vi "Robo Garra - Apres13.05.vi"   [LabVIEW 2016]
uses:
  <vilib>/NXT/Subs/LVHSConnector.ctl
  <vilib>/NXT/LegoClasses/BrickReference/BrickReference.lvclass
  <vilib>/NXT/Block Support/NXT_OutputPort.ctl
  <vilib>/NXT/Block Support/NXT_InputPort.ctl
  <vilib>/NXT/Block Support/NXT_ButtonSelector.ctl
  <vilib>/NXT/Dual Mode Library/Waits/Wait_Num.vi
  <vilib>/NXT/NXTIO Xnodes/NXTIONodeSubVIs/NXTMoveMotors.vi
  <vilib>/NXT/NXTIO Xnodes/NXTIONodeSubVIs/NXTStopMotors.vi
  <vilib>/NXT/Dual Mode Library/Sensors/EV3_Color_Reflect.vi
  <vilib>/NXT/Dual Mode Library/Sound/Tone.vi
  <vilib>/NXT/Dual Mode Library/Sensors/EV3_Ultrasonic_CM.vi
  <vilib>/NXT/Dual Mode Library/Sensors/readNXTButton.vi
  <vilib>/NXT/NXTIO Xnodes/AddressXNode/NXTIOAddress.xnode
  <vilib>/NXT/NXTIO Xnodes/NXTIOXNode/NXTIO.xnode
types:
  T1 = typedef "LVHSConnector.ctl" = refnum<class "BrickReference.lvclass">
  T2 = typedef "NXT_OutputPort.ctl" = u8
  T3 = typedef "NXT_ButtonSelector.ctl" = u16
  T4 = typedef "NXT_InputPort.ctl" = u32
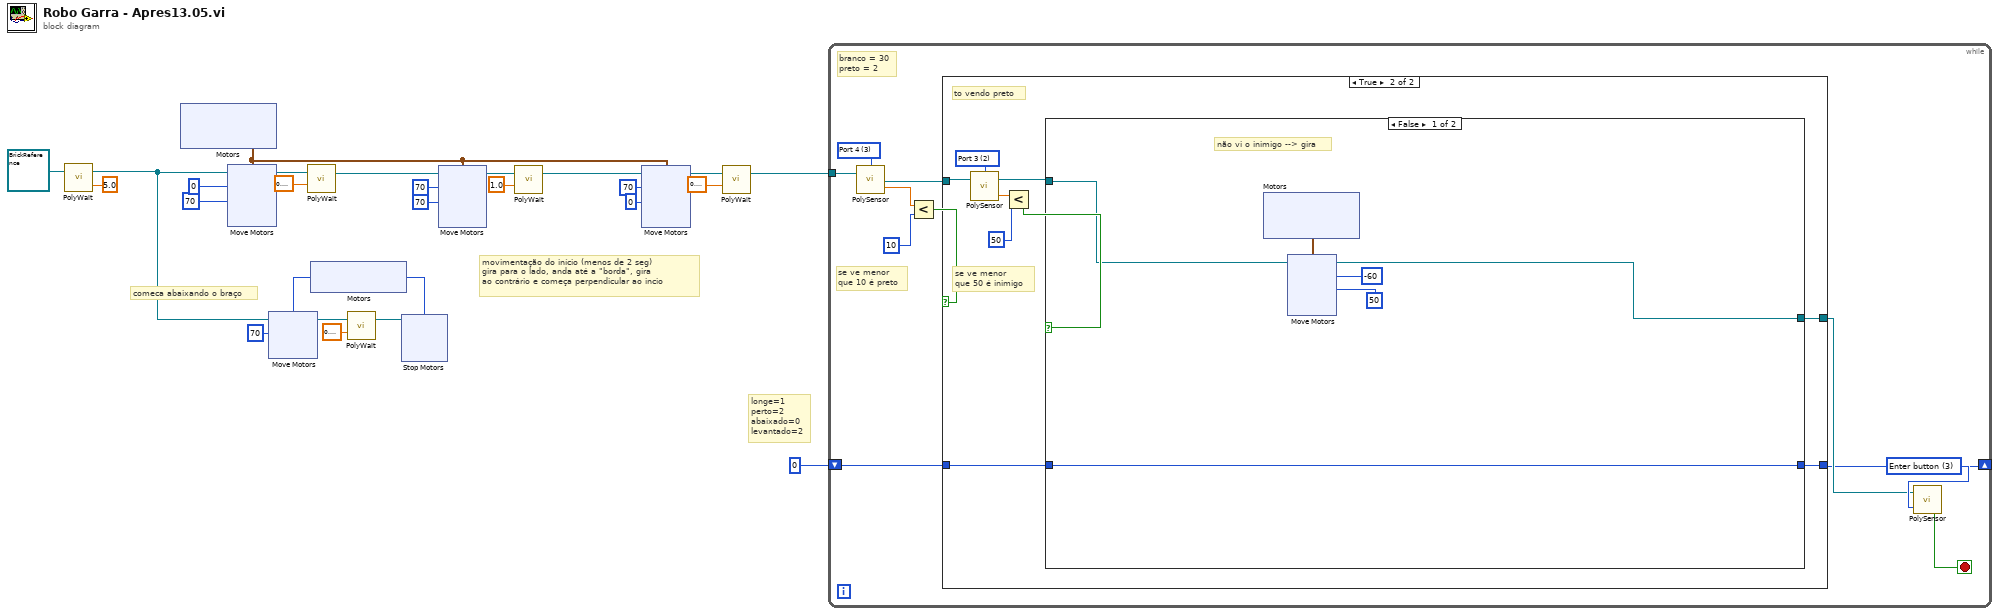
[diagram p0: block diagram]
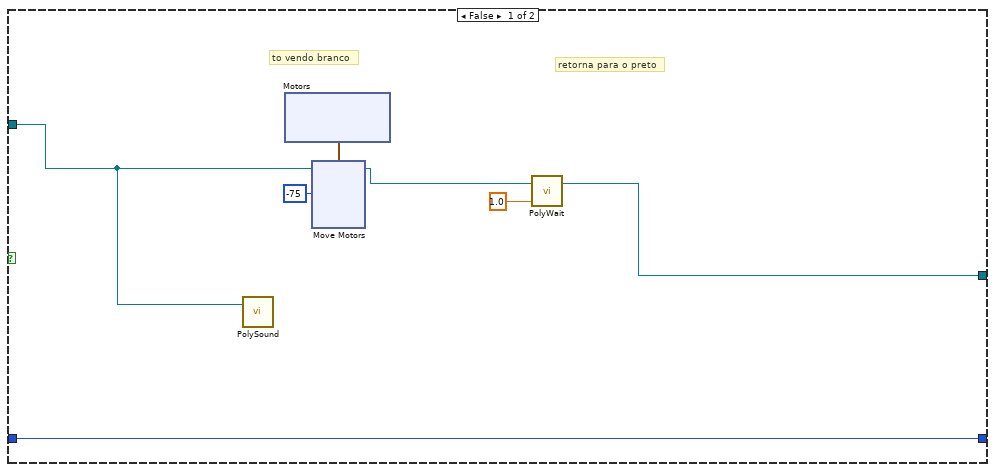
[diagram p2: hidden frame]
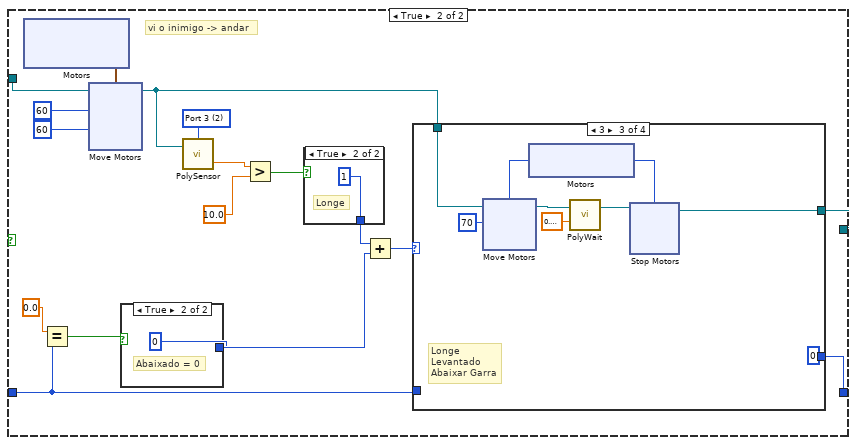
[diagram p3: hidden frame]
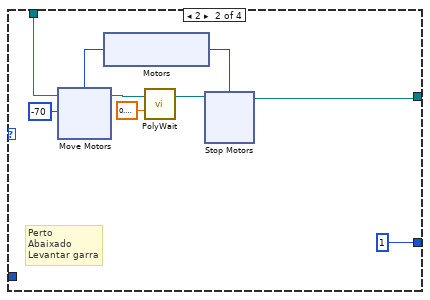
[diagram p5: hidden frame]
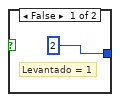
[diagram p7: hidden frame]
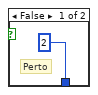
[diagram p8: hidden frame]
diagram:
  # "movimentação do início (menos de 2 seg)\ngira para o lado, anda até a \"borda\", gira \nao contrário e começa perpendicular ao incio"
  # "comeca abaixando o braço"
  # "longe=1\nperto=2\nabaixado=0\nlevantado=2"
  n1 = call-poly <vilib>:"PolyWait.vi"("Time (1 sec)"=sgl 5.0, "NXT/EV3"=T1 refnum ("y")) -> ("NXT/EV3"=w15:T1)  [unwired: 2 in]
  n2 = xnode "Motors"() -> ("Motor"=w7:cluster{"Port":T2, "Port":T2})
  n3 = xnode "Move Motors"("Power/Speed 2"=i8 70, "Power/Speed 1"=i8 0, "Motors"=w7, "NXT/EV3"=w15) -> ("NXT/EV3"=w13:T1)
  n4 = call-poly <vilib>:"PolyWait.vi"("Time (1 sec)"=sgl 0.3, "NXT/EV3"=w13) -> ("NXT/EV3"=w3:T1)  [unwired: 2 in]
  n5 = xnode "Motors"() -> ("Motor"=w19:T2)
  n6 = xnode "Move Motors"("Power/Speed 1"=i8 70, "Motors"=w19, "NXT/EV3"=w15) -> ("NXT/EV3"=w21:T1)
  n7 = call-poly <vilib>:"PolyWait.vi"("Time (1 sec)"=sgl 0.3, "NXT/EV3"=w21) -> ("NXT/EV3"=w22:T1)  [unwired: 2 in]
  n8 = xnode "Stop Motors"("Motors"=w19, "NXT/EV3"=w22) -> ()  [unwired: 1 out]
  n9 = xnode "Move Motors"("Power/Speed 2"=i8 70, "Power/Speed 1"=i8 70, "Motors"=w7, "NXT/EV3"=w3) -> ("NXT/EV3"=w10:T1)
  n10 = call-poly <vilib>:"PolyWait.vi"("Time (1 sec)"=sgl 1.0, "NXT/EV3"=w10) -> ("NXT/EV3"=w2:T1)  [unwired: 2 in]
  n11 = xnode "Move Motors"("Power/Speed 2"=i8 0, "Power/Speed 1"=i8 70, "Motors"=w7, "NXT/EV3"=w2) -> ("NXT/EV3"=w4:T1)
  n12 = call-poly <vilib>:"PolyWait.vi"("Time (1 sec)"=sgl 0.3, "NXT/EV3"=w4) -> ("NXT/EV3"=w1:T1)  [unwired: 2 in]
  n13 = while {
    tunnel: w1 -> [w35]
    shift-right: [w28] -> _
    shift-left: 0 -> [w32]
    stop <- w30 stop-if-true
    w31 = T3 3 items=["Enter button"=3, "Left button"=2, "Right button"=1, "Up Button"=4, "Down Button"=5] ("Button (Enter button)")
    w33 = T4 3 items=["Port 1", "Port 2", "Port 3", "Port 4"] ("Port (Port 1)")
    # "se ve menor \nque 10 é preto"
    # "branco = 30\npreto = 2"
    n14 = call-poly <vilib>:"PolySensor.vi"("NXT/EV3"=w35, "Port (Port 1)"=w33) -> ("Scaled Value"=w36:sgl, "NXT/EV3"=w34:T1)  [unwired: 1 in]
    n15 = Less?(x=w36, y=10) -> (x < y?=w27:bool)
    n16 = case shown="True" w27 {
      tunnel: w34 -> [w37 w61]
      tunnel: w32 -> [w38 w58]
      tunnel: [w39 w57] -> w29
      tunnel: [w38 w56] -> w28
      frame False {
        w42 = i8 -75 ("Power/Speed 2")
        # "retorna para o preto"
        # "to vendo branco"
        n17 = call-poly <vilib>:"PolySound.vi"("NXT/EV3"=w37) -> ()  [unwired: 3 in, 1 out]
        n18 = xnode "Motors"() -> ("Motor"=w43:cluster{"Port":T2, "Port":T2})
        n19 = xnode "Move Motors"("Power/Speed 2"=w42, "Power/Speed 1"=w42, "Motors"=w43, "NXT/EV3"=w37) -> ("NXT/EV3"=w40:T1)
        n20 = call-poly <vilib>:"PolyWait.vi"("Time (1 sec)"=sgl 1.0, "NXT/EV3"=w40) -> ("NXT/EV3"=w39:T1)  [unwired: 2 in]
      }
      frame True {
        w60 = T4 2 items=["Port 1", "Port 2", "Port 3", "Port 4"] ("Port (Port 1)")
        # "to vendo preto"
        # "se ve menor \nque 50 é inimigo"
        n21 = call-poly <vilib>:"PolySensor.vi"("NXT/EV3"=w61, "Port (Port 1)"=w60) -> ("Centimeters"=w54:sgl, "NXT/EV3"=w59:T1)  [unwired: 1 in]
        n22 = Less?(x=w54, y=50) -> (x < y?=w53:bool)
        n23 = case shown="False" w53 {
          tunnel: w59 -> [w65 w78]
          tunnel: w58 -> [w63 w77]
          tunnel: [w64 w82] -> w57
          tunnel: [w63 w81] -> w56
          frame False {
            # "não vi o inimigo --> gira"
            n24 = xnode "Motors"() -> ("Motor"=w66:cluster{"Port":T2, "Port":T2})
            n25 = xnode "Move Motors"("Power/Speed 2"=i8 50, "Power/Speed 1"=i8 -60 ("Power/Speed 2"), "Motors"=w66, "NXT/EV3"=w65) -> ("NXT/EV3"=w64:T1)
          }
          frame True {
            w90 = T4 2 items=["Port 1", "Port 2", "Port 3", "Port 4"] ("Port (Port 1)")
            # "vi o inimigo -> andar"
            n26 = xnode "Motors"() -> ("Motor"=w93:cluster{"Port":T2, "Port":T2})
            n27 = Equal?(x=0.0, y=w77) -> (x = y?=w84:bool)
            n28 = xnode "Move Motors"("Power/Speed 2"=i8 60, "Power/Speed 1"=i8 60, "Motors"=w93, "NXT/EV3"=w78) -> ("NXT/EV3"=w88:T1)
            n29 = case shown="True" w84 {
              tunnel: [2 0] -> w85
              frame False {
                # "Levantado = 1"
              }
              frame True {
                # "Abaixado = 0"
              }
            }
            n30 = call-poly <vilib>:"PolySensor.vi"("NXT/EV3"=w88, "Port (Port 1)"=w90) -> ("Centimeters"=w91:sgl)  [unwired: 1 in, 1 out]
            n31 = Greater?(x=w91, y=sgl 10.0) -> (0:w89:bool)
            n32 = case shown="True" w89 {
              tunnel: [2 1] -> w86
              frame False {
                # "Perto"
              }
              frame True {
                # "Longe"
              }
            }
            n33 = Add(x=w86, y=w85) -> (x+y=w83:i32)
            n34 = case shown="3" w83 {
              tunnel: w88 -> [w95 w96 w118 w139]
              tunnel: [w95 w97 w117 w139] -> w82
              tunnel: [w94 1 0 w138] -> w81
              tunnel: w77 -> [w94 _ _ w138]
              frame 1, Default {
                # "Longe\nAbaixado\nAnda"
              }
              frame 2 {
                # "Perto\nAbaixado\nLevantar garra"
                n35 = xnode "Motors"() -> ("Motor"=w102:T2)
                n36 = xnode "Move Motors"("Power/Speed 1"=i8 -70, "Motors"=w102, "NXT/EV3"=w96) -> ("NXT/EV3"=w100:T1)
                n37 = call-poly <vilib>:"PolyWait.vi"("Time (1 sec)"=sgl 0.3, "NXT/EV3"=w100) -> ("NXT/EV3"=w99:T1)  [unwired: 2 in]
                n38 = xnode "Stop Motors"("Motors"=w102, "NXT/EV3"=w99) -> ("NXT/EV3"=w97:T1)
              }
              frame 3 {
                # "Longe\nLevantado\nAbaixar Garra"
                n39 = xnode "Motors"() -> ("Motor"=w119:T2)
                n40 = xnode "Move Motors"("Power/Speed 1"=i8 70, "Motors"=w119, "NXT/EV3"=w118) -> ("NXT/EV3"=w121:T1)
                n41 = call-poly <vilib>:"PolyWait.vi"("Time (1 sec)"=sgl 0.3, "NXT/EV3"=w121) -> ("NXT/EV3"=w122:T1)  [unwired: 2 in]
                n42 = xnode "Stop Motors"("Motors"=w119, "NXT/EV3"=w122) -> ("NXT/EV3"=w117:T1)
              }
              frame 4 {
                # "Perto\nLevantado\nAnda"
              }
            }
          }
        }
      }
    }
    n43 = call-poly <vilib>:"PolySensor.vi"("Button (Enter button)"=w31, "NXT/EV3"=w29) -> ("Yes/No"=w30:bool)  [unwired: 1 in, 1 out]
  }
